vi "Protocol Write.vi"(8 "error in":errorcluster, 9 "timeout":i32=10000, 10 "data":u8[](array[numeric]), 11 "protocol layer in":refnum<class "TCP Slave.lvclass">) -> (0 "error out":errorcluster, 1 "Timed out":bool, 3 "protocol layer out":refnum<class "TCP Slave.lvclass">)   [LabVIEW 2021]
doc: "Writes to the established TCP connection stored in the class."
uses:
  TCP Slave.lvclass
  TCP Slave.lvclass/TCP Slave.ctl
  <vilib>/Utility/error.llb/Clear Errors.vi
  TCP Shared Components/TCP Shared Components.lvlib
  D:/my_projects/projects/Algorithms/Labview/21/Modbus_v121c/Network Protocol/Network Slave/Network Slave.lvclass
  D:/my_projects/projects/Algorithms/Labview/21/Modbus_v121c/Network Protocol/Network Protocol.lvclass
  D:/my_projects/projects/Algorithms/Labview/21/Modbus_v121c/Network Protocol/Network Slave/TCP/TCP Slave.lvclass
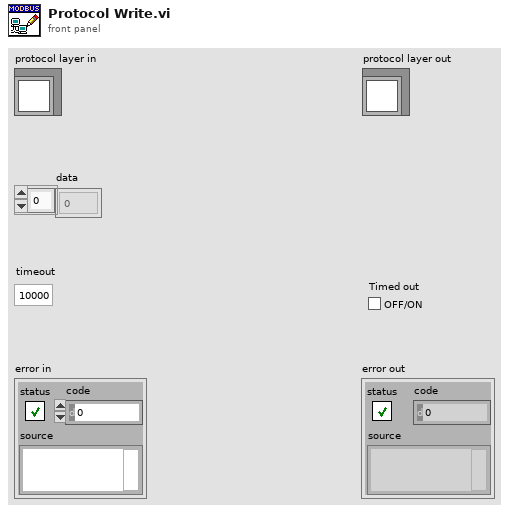
[diagram p1: front panel]
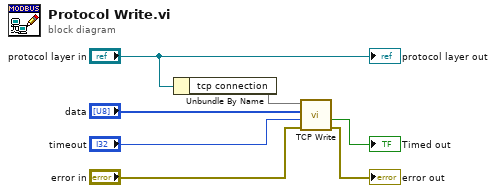
[diagram p0: block diagram]
diagram:
  n1 = Unbundle By Name("protocol layer in") -> ("tcp connection"=w5)
  n2 = call "TCP Write.vi"("error in"="error in", "timeout"="timeout", "data"="data", "connection ID"=w5) -> ("error out"=→"error out":errorcluster, "timed out?"=→"Timed out":bool)  [unwired: 6 in]
  "protocol layer out" <- "protocol layer in"
